vi "Init.vi"(3 "Container State":T3, 4 "Previous State":variant=variant(cluster{"Type":enum16{"Sine", "Triangle", "Saw Tooth", "Square"}, "Periods":dbl, "Points":dbl, "Offset":dbl, "Amplitdue":dbl, "Starting Phase":dbl, "Show Axes":bool, "Show Y=0":bool} {"Type"=enum."Sine", "Periods"=0.0, "Points"=0.0, "Offset"=0.0, "Amplitdue"=0.0, "Starting Phase"=0.0, "Show Axes"=FALSE, "Show Y=0"=FALSE}), 5 "Previous Version":T2) -> (2 "Current State":T1)   [LabVIEW 2012, in "Waveform Control.xctl"]
uses:
  Waveform Control.xctl
  Controls/Waveform State.ctl
  subvis/FP Controls.ctl
  subvis/Function Types.ctl
  <vilib>/_xctls/Container State.ctl
  <vilib>/_xctls/Version.ctl
  Controls/State.ctl
  Controls/Volatile State Ops.ctl
  <vilib>/_xctls/XControlSupport.lvlib
panel:
  in  "Default Indicator State":T4={"Show Axes"=FALSE, "Show Y=0"=TRUE, "Controls"={"Type"=enum."Sine", "Periods"=0.0, "Points"=0, "Offset"=0.0, "Amplitdue"=0.0, "Starting Phase"=0.0, "func"=""}, "Show Current Location"=TRUE, "Current Location"=0, "dt"=0.0, "t0"=timestamp(0 s since 1904-01-01), "Amplitude Format String"="%_3p"} {"Controls"."Points" format="%_3p"}
  in  "Default Control State":T4={"Show Axes"=FALSE, "Show Y=0"=TRUE, "Controls"={"Type"=enum."Sine", "Periods"=0.0, "Points"=0, "Offset"=0.0, "Amplitdue"=0.0, "Starting Phase"=0.0, "func"=""}, "Show Current Location"=TRUE, "Current Location"=0, "dt"=0.0, "t0"=timestamp(0 s since 1904-01-01), "Amplitude Format String"="%_3p"} {"Controls"."Points" format="%_3p"}
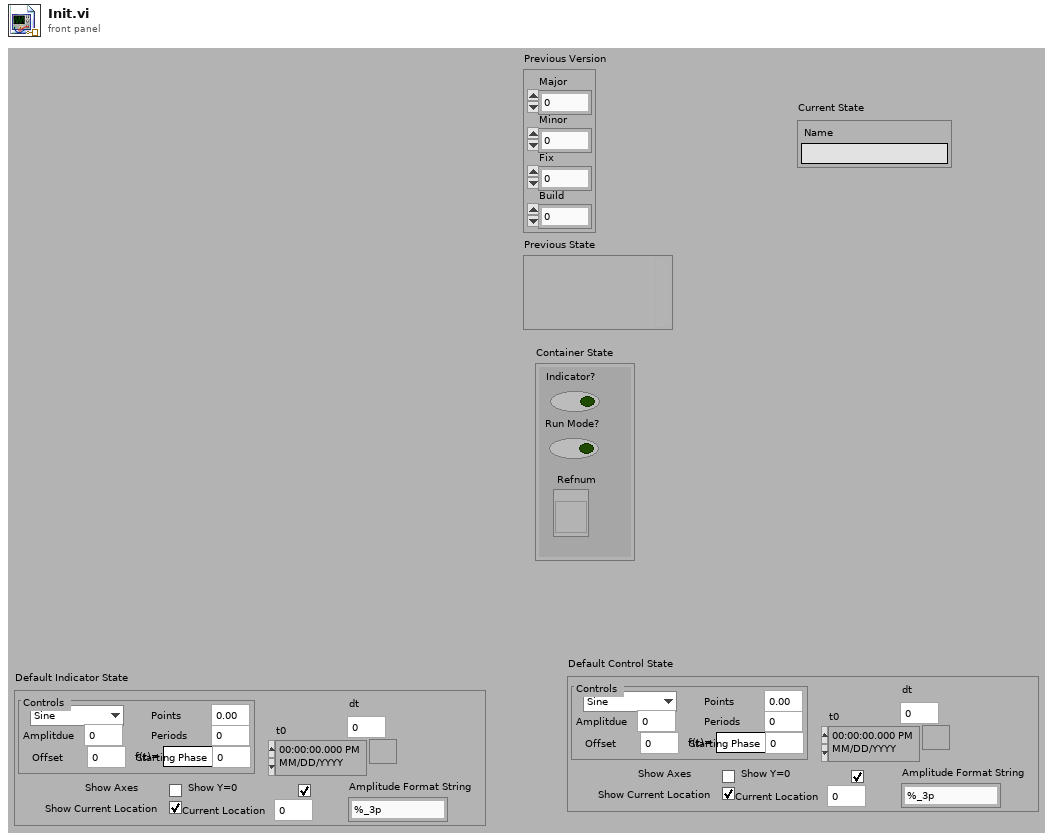
[diagram p1: front panel]
types:
  T1 = typedef "Waveform Control.xctl/State.ctl" = cluster{"Name":string}
  T2 = typedef "XControlSupport.lvlib/Version.ctl" = cluster{"Major":u16, "Minor":u16, "Fix":u16, "Build":u16}
  T3 = typedef "XControlSupport.lvlib/Container State.ctl" = cluster{"Indicator?":bool, "Run Mode?":bool, " Refnum":refnum<vi>}
  T4 = typedef "Waveform Control.xctl/Waveform State.ctl" = cluster{"Show Axes":bool, "Show Y=0":bool, "Controls":T5, "Show Current Location":bool, "Current Location":i32, "dt":dbl, "t0":timestamp, "Amplitude Format String":string}
  T5 = typedef "Waveform Control.xctl/FP Controls.ctl" = cluster{"Type":T6, "Periods":dbl, "Points":i32, "Offset":dbl, "Amplitdue":dbl, "Starting Phase":dbl, "func":string}
  T6 = typedef "Waveform Control.xctl/Function Types.ctl" = enum16{"Level", "Sine", "Triangle", "Ramp", "Saw Tooth", "Square", "Function"}
  T7 = typedef "Waveform Control.xctl/Volatile State Ops.ctl" = enum16{"Read", "Write", "Update State from Data"}
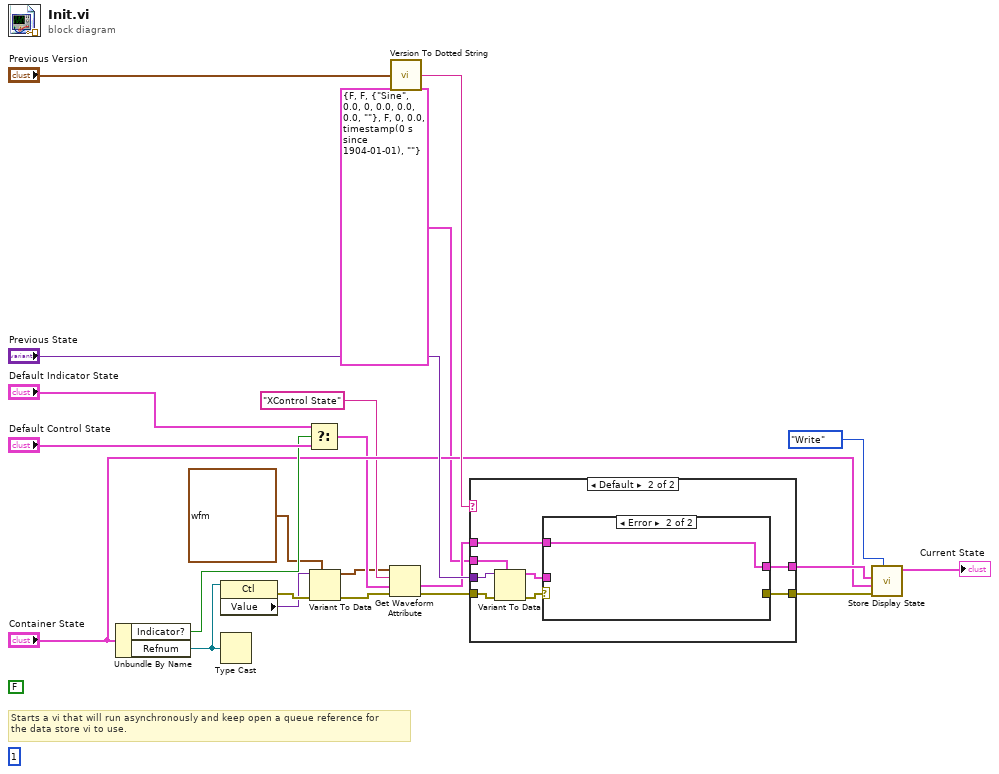
[diagram p0: block diagram]
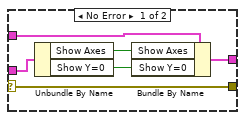
[diagram p3: hidden frame]
diagram:
  (unwired) FALSE ("ignore previous (F)")
  (unwired) 1 ("max queue size (-1, unlimited)")
  # "Starts a vi that will run asynchronously and keep open a queue reference for\nthe data store vi to use."
  n1 = Unbundle By Name("Container State") -> ("Indicator?"=w19:bool, "Refnum"=w3:refnum<vi>)
  n2 = property class="Ctl"(reference=w3) -> (error out=w8:errorcluster, "Value"=w7:variant)  [unwired: 1 in, 1 out]
  n3 = Type Cast(x=w3) -> ()  [unwired: 2 out]
  n4 = Select(t="Default Indicator State", s=w19, f="Default Control State") -> (s? t:f=w11:T4)
  n5 = Variant To Data(error in=w8, type=waveform(dbl) {"t0"=timestamp(0 s since 1904-01-01), "dt"=1.0, "Y"=[]} ("waveform"), Variant=w7) -> (data=w5:waveform(dbl), error out=w6:errorcluster)
  n6 = Get Waveform Attribute(4:w6, 5:w11, 6:"XControl State" ("name"), 7:w5) -> (0:w9:errorcluster, 1:w10:T4)  [unwired: 2 out]
  n7 = call <vilib>:"Version To Dotted String.vi"("Version"="Previous Version") -> ("String Version"=w17:string)
  n8 = case shown="Default" w17 {
    tunnel: "Previous State" -> [_ w31]
    tunnel: [w23 w27] -> w16
    tunnel: w10 -> [w23 w28]
    tunnel: [_ w26] -> w1
    tunnel: T4 {"Show Axes"=FALSE, "Show Y=0"=FALSE, "Controls"={"Type"=enum."Sine", "Periods"=0.0, "Points"=0, "Offset"=0.0, "Amplitdue"=0.0, "Starting Phase"=0.0, "func"=""}, "Show Current Location"=FALSE, "Current Location"=0, "dt"=0.0, "t0"=timestamp(0 s since 1904-01-01), "Amplitude Format String"=""} ("Waveform State Out") -> [_ w25]
    tunnel: w9 -> [_ w24]
    frame "0.0.0.0" {
    }
    frame Default {
      n9 = Variant To Data(error in=w24, type=w25, Variant=w31) -> (data=w29:T4, error out=w30:errorcluster)
      n10 = case shown="Error" w30 {
        selector: w30 -> [w37 _]
        tunnel: w29 -> [w35 _]
        tunnel: [w34 w38] -> w27
        tunnel: w28 -> [w36 w38]
        tunnel: [w37 _] -> w26
        frame No Error {
          n11 = Unbundle By Name(w35) -> ("Show Axes"=w33:bool, "Show Y=0"=w32:bool)
          n12 = Bundle By Name(cluster=w36, "Show Axes"=w33, "Show Y=0"=w32) -> (w34:T4)
        }
        frame Error {
        }
      }
    }
  }
  n13 = call "Store Display State.vi"("Operation In"=Volatile_State_Ops."Write", "Error In (no Error) In"=w1, "Container State In"="Container State", "Waveform State In"=w16) -> ("Display State Out"=→"Current State":T1)  [unwired: 2 in, 5 out]
